vi "ROS_Master_unregisterPubSubReply.vi"(2 "PubSub":T1, 3 "error in":errorcluster) -> (1 "XML":string)   [LabVIEW 2015]
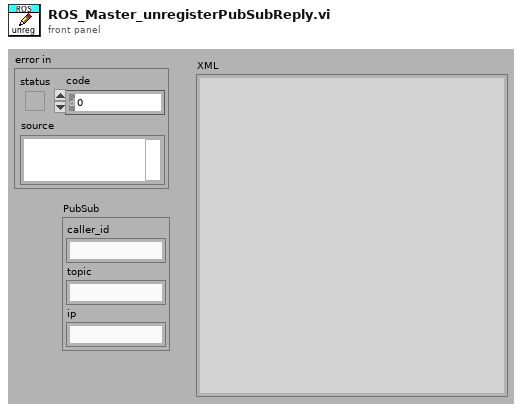
[diagram p1: front panel]
types:
  T1 = cluster{"caller_id":string, "topic":string, "ip":string}
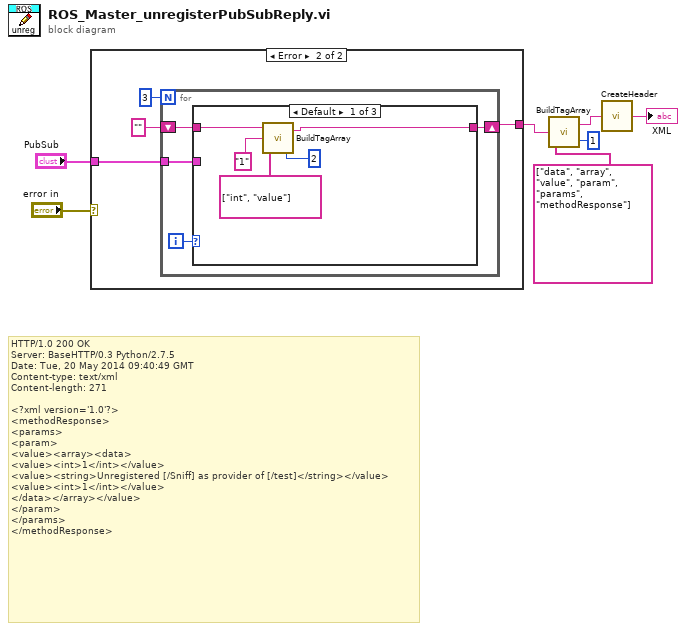
[diagram p0: block diagram]
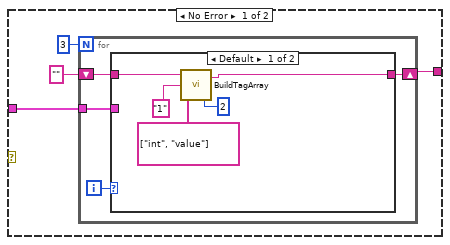
[diagram p2: hidden frame]
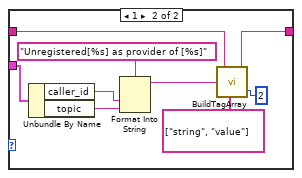
[diagram p3: hidden frame]
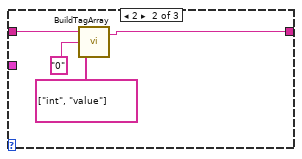
[diagram p4: hidden frame]
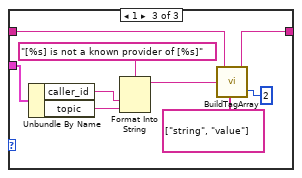
[diagram p5: hidden frame]
diagram:
  # "HTTP/1.0 200 OK\nServer: BaseHTTP/0.3 Python/2.7.5\nDate: Tue, 20 May 2014 09:40:49 GMT\nContent-type: text/xml\nContent-length: 271\n\n<?xml version='1.0'?>\n<methodResponse>\n<params>\n<param>\n<value><array><data>\n<value><int>1</int></value>\n<value><string>Unregistered [/Sniff] as provider of [/test]</string></value>\n<value><int>1</int></value>\n</data></array></value>\n</param>\n</params>\n</methodResponse>"
  n1 = case shown="Error" "error in" {
    tunnel: "PubSub" -> [w9 w31]
    tunnel: [w8 w30] -> w4
    frame No Error {
      n2 = for {
        N: 3 -> [_]
        shift-right: [w12] -> w8
        shift-left: "" ("caller_id") -> [w14]
        tunnel: w9 -> [w13]
        i -> [w15]
        n3 = case shown="Default" w15 {
          tunnel: w14 -> [w18 w23]
          tunnel: w13 -> [_ w28]
          tunnel: [w17 w22] -> w12
          frame Default {
            n4 = call "BuildTagArray.vi"("Indent"=i8 2, "tags"=string[] ["int", "value"], "value"="1", "string in"=w18) -> ("string out"=w17:string)
          }
          frame 1 {
            n5 = Unbundle By Name(w28) -> ("caller_id"=w26:string, "topic"=w25:string)
            n6 = Format Into String(format string="Unregistered[%s] as provider of [%s]", w26, w25) -> (resulting string=w24:string)  [unwired: 2 in, 1 out]
            n7 = call "BuildTagArray.vi"("Indent"=i8 2, "tags"=string[] ["string", "value"], "value"=w24, "string in"=w23) -> ("string out"=w22:string)
          }
        }
      }
    }
    frame Error {
      n8 = for {
        N: 3 -> [_]
        shift-right: [w34] -> w30
        shift-left: "" ("caller_id") -> [w36]
        tunnel: w31 -> [w35]
        i -> [w37]
        n9 = case shown="Default" w37 {
          tunnel: w36 -> [w40 w44 w49]
          tunnel: w35 -> [_ _ w54]
          tunnel: [w39 w43 w48] -> w34
          frame Default {
            n10 = call "BuildTagArray.vi"("Indent"=i8 2, "tags"=string[] ["int", "value"], "value"="1", "string in"=w40) -> ("string out"=w39:string)
          }
          frame 2 {
            n11 = call "BuildTagArray.vi"("tags"=string[] ["int", "value"], "value"="0", "string in"=w44) -> ("string out"=w43:string)  [unwired: 1 in]
          }
          frame 1 {
            n12 = Unbundle By Name(w54) -> ("caller_id"=w52:string, "topic"=w51:string)
            n13 = Format Into String(format string="[%s] is not a known provider of [%s]", w52, w51) -> (resulting string=w50:string)  [unwired: 2 in, 1 out]
            n14 = call "BuildTagArray.vi"("Indent"=i8 2, "tags"=string[] ["string", "value"], "value"=w50, "string in"=w49) -> ("string out"=w48:string)
          }
        }
      }
    }
  }
  n15 = call "BuildTagArray.vi"("Indent"=i8 1, "tags"=string[] ["data", "array", "value", "param", "params", "methodResponse"], "value"=w4) -> ("string out"=w3:string)  [unwired: 1 in]
  n16 = call "CreateHeader.vi"("Content"=w3) -> ("XML"=→"XML":string)
